vi "Update Cache.vi"(9 "Classes":refnum<class>[](array[class]), 10 "Paths":path[](array[path]), 11 "Class Loader in":refnum<class "Class Loader.lvclass">) -> (3 "Class Loader out":refnum<class "Class Loader.lvclass">)   [LabVIEW 2023, in "Class Loader.lvlib" / "Class Loader.lvclass"]
uses:
  Class Loader.lvclass
  Class Loader.lvclass/Class Loader.ctl
  <vilib>/Utility/miscctls.llb/LVMapReplaceAction.ctl
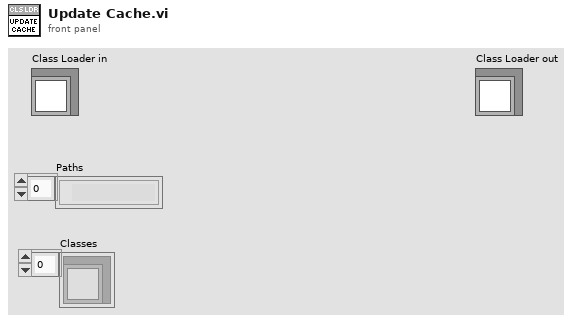
[diagram p1: front panel]
types:
  T1 = typedef "LVMapReplaceAction.ctl" = enum32{"Modify Entry only if found", "Add or Modify Entry", "Delete Entry"}
  T2 = typedef "Class Loader.lvlib/Class Loader.lvclass/Classes Cache Map.ctl" = map{path, refnum<class>}
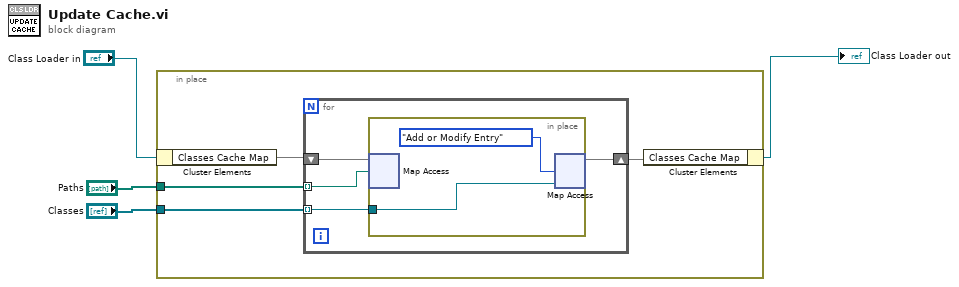
[diagram p0: block diagram]
diagram:
  n1 = in-place {
    in-place-border: "Paths" -> [w8]
    in-place-border: "Classes" -> [w7]
    n2 = in-place-cluster #1("Class Loader in") -> ("Classes Cache Map"=w6:T2)
    n3 = for {
      shift-right: [w10] -> w5
      shift-left: w6 -> [w9]
      tunnel: w8 -> [w12] mode=indexing
      tunnel: w7 -> [w11] mode=indexing
      n4 = in-place {
        in-place-border: w11 -> [w13]
        n5 = in-place-map #2(w9, w12) -> ()  [unwired: 1 in, 2 out]
        n6 = in-place-map #2(w13, LVMapReplaceAction."Add or Modify Entry" ("action")) -> (w10:T2)  [unwired: 2 out]
      }
    }
    n7 = in-place-cluster #1("Classes Cache Map"=w5) -> (→"Class Loader out":refnum<class "Class Loader.lvclass">)
  }
